vi "PreBuildTest(Fail).vi"(8 "error in (no error)":errorcluster) -> (0 "error out":errorcluster)   [LabVIEW 2013]
uses:
  classes/Test Suite/Test Suite.lvclass
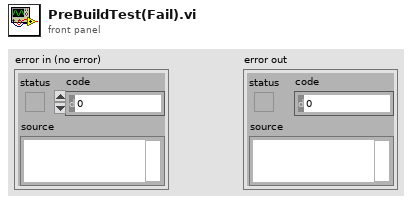
[diagram p1: front panel]
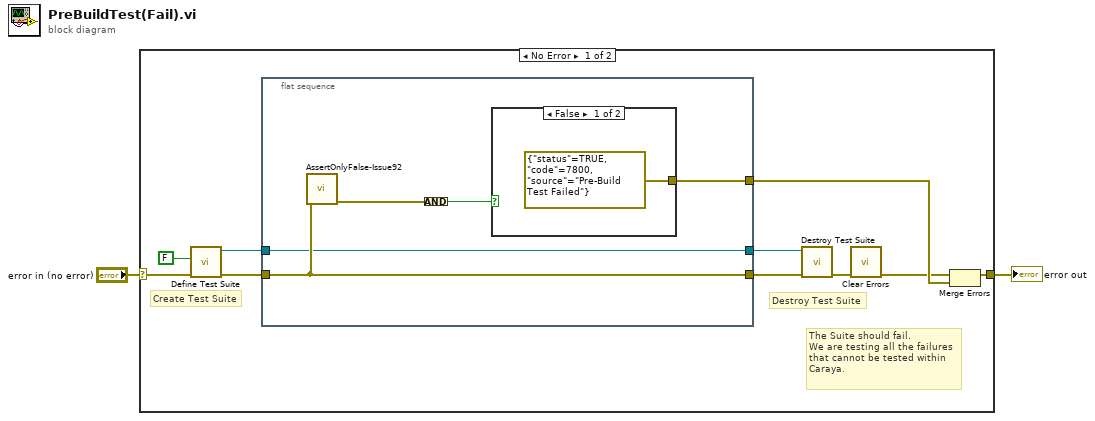
[diagram p0: block diagram]
diagram:
  n1 = case shown="No Error" "error in (no error)" {
    selector: "error in (no error)" -> [w9 w19]
    tunnel: [w5 w19] -> w1
    frame No Error {
      # "The Suite should fail.\nWe are testing all the failures\nthat cannot be tested within\nCaraya."
      # "Destroy Test Suite"
      # "Create Test Suite"
      n2 = call "Define Test Suite.vi"("error in (no error)"=w9, "Interactive"=FALSE) -> ("error out"=w12:errorcluster, "Test Suite"=w8:refnum<class "Test Suite.lvclass">)  [unwired: 8 in]
      n3 = flat-sequence {
        tunnel: w12 -> [w17]
        tunnel: [w17] -> w11
        tunnel: w8 -> [w16]
        tunnel: [w16] -> w7
        tunnel: [w13] -> w6
        frame #0 {
          n4 = call "AssertOnlyFalse-Issue92.vi"("error in"=w17) -> ("error out"=w15:errorcluster)  [unwired: 10 in]
          n5 = Compound Arithmetic op=AND(w15) -> (w14:bool)
          n6 = case shown="False" w14 {
            tunnel: [errorcluster {"status"=TRUE, "code"=7800, "source"="Pre-Build Test Failed"} ("error constant") _] -> w13
            frame False {
            }
            frame True {
              # "FAILURE DETECTED\nSUCCESSFULLY"
            }
          }
        }
      }
      n7 = call-dynamic "Destroy Test Suite.vi"("error in (no error)"=w11, "Test Suite in"=w7) -> ("error out"=w4:errorcluster)  [unwired: 9 in]
      n8 = call <vilib>:"Clear Errors.vi"("error in (no error)"=w4) -> ("error out"=w3:errorcluster)  [unwired: 6 in]
      n9 = Merge Errors(w3, w6) -> (w5:errorcluster)
    }
    frame Error {
    }
  }
  "error out" <- w1
